vi "Read Page Orientaion.vi"(0 "PdfReader ref":refnum<k24>, 5 "PdfReader page number":i32, 7 "Actual Page number":i32, 9 "Pages dimensions [ ] IN":T1[](array[typedef]) {"Page Size" items=["Custom", "LETTER", "NOTE", "LEGAL", "TABLOID", "EXECUTIVE", "POSTCARD", "A0", "A1", "A2", "A3", "A4", "A5", "A6", "A7", "A8", "A9", "A10", "B0", "B1", "B2", "B3", "B4", "B5", "B6", "B7", "B8", "B9", "B10", "ARCH_E", "ARCH_D", "ARCH_C", "ARCH_B", "ARCH_A", "FLSA", "FLSE", "HALFLETTER", "_11X17", "ID_1", "ID_2", "ID_3", "LEDGER", "CROWN_QUARTO", "LARGE_CROWN_QUARTO", "DEMY_QUARTO", "ROYAL_QUARTO", "CROWN_OCTAVO", "LARGE_CROWN_OCTAVO", "DEMY_OCTAVO", "ROYAL_OCTAVO", "SMALL_PAPERBACK", "PENGUIN_SMALL_PAPERBACK", "PENGUIN_LARGE_PAPERBACK"]}, 11 "error in (no error)":errorcluster) -> (4 "PdfReader ref duplicate":refnum<k24>, 10 "Pages dimensions OUT [ ]":T1[](array[typedef]) {"Page Size" items=["Custom", "LETTER", "NOTE", "LEGAL", "TABLOID", "EXECUTIVE", "POSTCARD", "A0", "A1", "A2", "A3", "A4", "A5", "A6", "A7", "A8", "A9", "A10", "B0", "B1", "B2", "B3", "B4", "B5", "B6", "B7", "B8", "B9", "B10", "ARCH_E", "ARCH_D", "ARCH_C", "ARCH_B", "ARCH_A", "FLSA", "FLSE", "HALFLETTER", "_11X17", "ID_1", "ID_2", "ID_3", "LEDGER", "CROWN_QUARTO", "LARGE_CROWN_QUARTO", "DEMY_QUARTO", "ROYAL_QUARTO", "CROWN_OCTAVO", "LARGE_CROWN_OCTAVO", "DEMY_OCTAVO", "ROYAL_OCTAVO", "SMALL_PAPERBACK", "PENGUIN_SMALL_PAPERBACK", "PENGUIN_LARGE_PAPERBACK"]}, 15 "error out":errorcluster)   [LabVIEW 2019]
doc: "Version 1.1\nDeveloped by Jean-Marc Simard\nCopyright © 2012, Exaprom Inc.\nAll rights reserved.\nLicense: BSD\n\nWith iTextSharp 4.1.6 (http://itextsharp.sourceforge.net)\nunder Mozilla Public License Version 1.1\n(http://www.mozilla.org/MPL/MPL-1.1.html)"
uses:
  <userlib>/Exaprom PDF/Controls/Page Controls/Page dimensions.ctl
  <userlib>/Exaprom PDF/Controls/Page Controls/Page size.ctl
  <userlib>/Exaprom PDF/Controls/Page Controls/Page Orientation.ctl
  C:/Program Files/National Instruments/LabVIEW 2019/user.lib/Exaprom PDF/DLL/itextsharp.dll
  DLL/itextsharp.dll
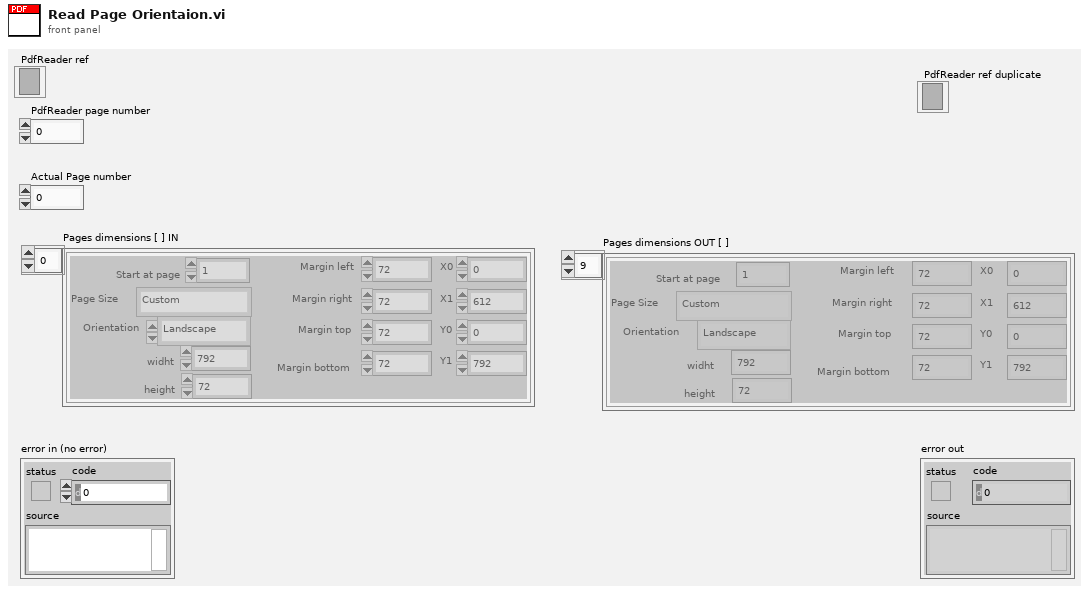
[diagram p1: front panel]
types:
  T1 = typedef "Page dimensions.ctl" = cluster{"Start at page":i32, "Page Size":T2, "Orientation":T3, "widht":sgl, "height":sgl, "Margin left":sgl, "Margin right":sgl, "Margin top":sgl, "Margin bottom":sgl, "X0":sgl, "X1":sgl, "Y0":sgl, "Y1":sgl}
  T2 = typedef "Page size.ctl" = i32
  T3 = typedef "Page Orientation.ctl" = enum16{"Portrait", "Landscape"}
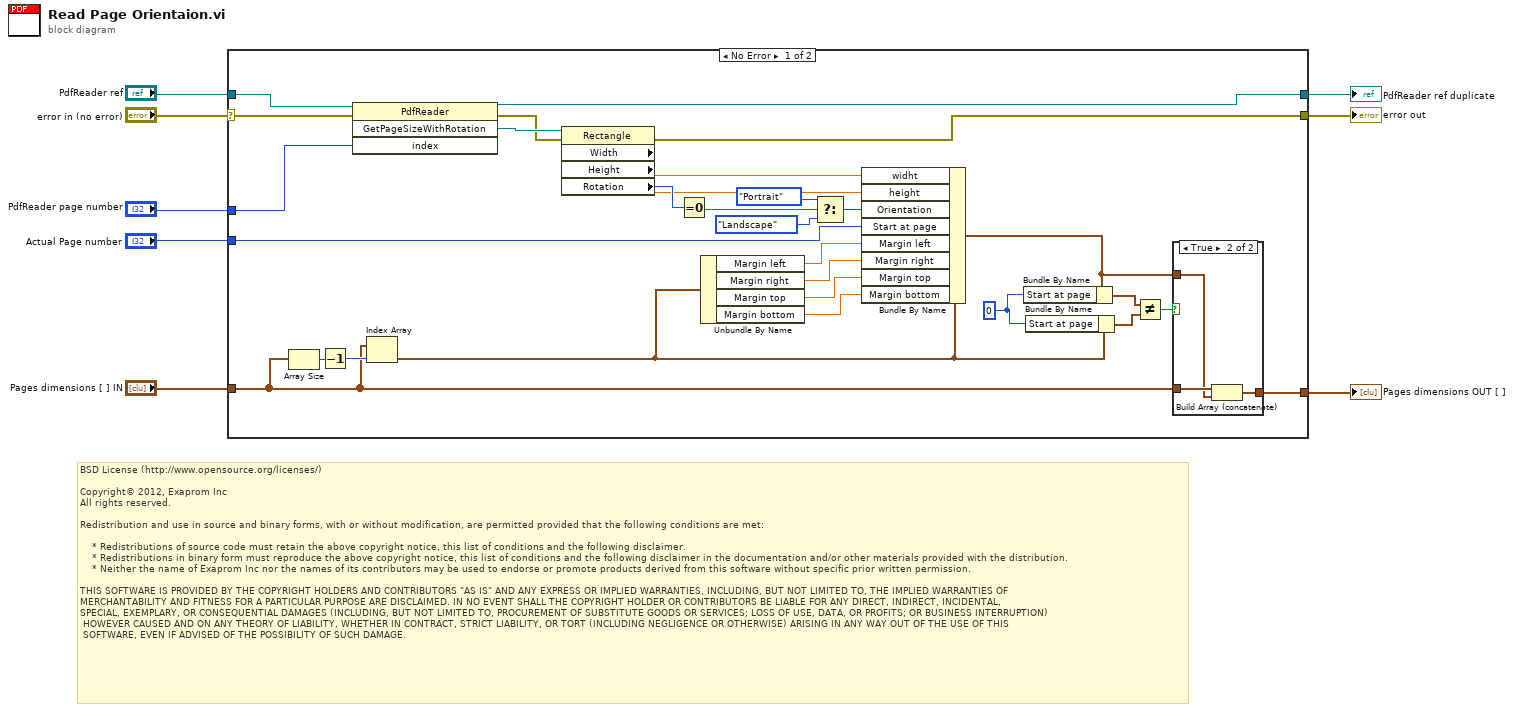
[diagram p0: block diagram]
diagram:
  # "BSD License (http://www.opensource.org/licenses/)\n\nCopyright© 2012, Exaprom Inc\nAll rights reserved.\n\nRedistribution and use in source and binary forms, with or without modification, are permitted provided that the following conditions are met:\n\n    * Redistributions of source code must retain the above copyright notice, this list of conditions and the following disclaimer.\n    * Redistributions in binary form must reproduce the above copyright notice, this list of conditions and the following disclaimer in the documentation and/or other materials provided with the distribution.\n    * Neither the name of Exaprom Inc nor the names of its contributors may be used to endorse or promote products derived from this software without specific prior written permission.\n\nTHIS SOFTWARE IS PROVIDED BY THE COPYRIGHT HOLDERS AND CONTRIBUTORS \"AS IS\" AND ANY EXPRESS OR IMPLIED WARRANTIES, INCLUDING, BUT NOT LIMITED TO, THE IMPLIED WARRANTIES OF \nMERCHANTABILITY AND FITNESS FOR A PARTICULAR PURPOSE ARE DISCLAIMED. IN NO EVENT SHALL THE COPYRIGHT HOLDER OR CONTRIBUTORS BE LIABLE FOR ANY DIRECT, INDIRECT, INCIDENTAL,\nSPECIAL, EXEMPLARY, OR CONSEQUENTIAL DAMAGES (INCLUDING, BUT NOT LIMITED TO, PROCUREMENT OF SUBSTITUTE GOODS OR SERVICES; LOSS OF USE, DATA, OR PROFITS; OR BUSINESS INTERRUPTION)\n HOWEVER CAUSED AND ON ANY THEORY OF LIABILITY, WHETHER IN CONTRACT, STRICT LIABILITY, OR TORT (INCLUDING NEGLIGENCE OR OTHERWISE) ARISING IN ANY WAY OUT OF THE USE OF THIS\n SOFTWARE, EVEN IF ADVISED OF THE POSSIBILITY OF SUCH DAMAGE."
  n1 = case shown="No Error" "error in (no error)" {
    selector: "error in (no error)" -> [w16 w44]
    tunnel: [w15 w44] -> w8
    tunnel: [w14 w42] -> w6
    tunnel: [w13 w43] -> w5
    tunnel: "Pages dimensions [ ] IN" -> [w12 w42]
    tunnel: "Actual Page number" -> [w11 _]
    tunnel: "PdfReader page number" -> [w10 _]
    tunnel: "PdfReader ref" -> [w9 w43]
    frame No Error {
      w30 = 0
      n2 = Array Size(array=w12) -> (size(s)=w36:i32)
      n3 = Decrement(x=w36) -> (x-1=w35:i32)
      n4 = invoke class="PdfReader" method="GetPageSizeWithRotation"(reference=w9, error in=w16, "index"=w10) -> (reference out=w13:refnum<k24>, error out=w17:errorcluster, "GetPageSizeWithRotation"=w18:refnum<k24>)  [unwired: 1 in, 1 out]
      n5 = Index Array(array=w12, index=w35) -> (element=w37:T1)
      n6 = property class="Rectangle"(reference=w18, error in=w17) -> (error out=w15:errorcluster, "Width"=w19:sgl, "Height"=w20:sgl, "Rotation"=w21:i32)  [unwired: 1 out]
      n7 = Equal To 0?(x=w21) -> (x = 0?=w22:bool)
      n8 = Unbundle By Name(w37) -> ("Margin left"=w26:sgl, "Margin right"=w27:sgl, "Margin top"=w28:sgl, "Margin bottom"=w29:sgl)
      n9 = Select(t=Page_Orientation."Portrait" ("Orientation"), s=w22, f=Page_Orientation."Landscape" ("Orientation")) -> (s? t:f=w25:T3)
      n10 = Bundle By Name(cluster=w37, "widht"=w19, "height"=w20, "Orientation"=w25, "Start at page"=w11, "Margin left"=w26, "Margin right"=w27, "Margin top"=w28, "Margin bottom"=w29) -> (w34:T1)
      n11 = Bundle By Name(cluster=w34, "Start at page"=w30) -> (w31:T1)
      n12 = Bundle By Name(cluster=w37, "Start at page"=w30) -> (w32:T1)
      n13 = Not Equal?(x=w31, y=w32) -> (x != y?=w33:bool)
      n14 = case shown="True" w33 {
        tunnel: w12 -> [w38 w41]
        tunnel: [w38 w40] -> w14
        tunnel: w34 -> [_ w39]
        frame False {
        }
        frame True {
          n15 = Build Array (concatenate)(w41, w39) -> (w40:T1[])
        }
      }
    }
    frame Error {
    }
  }
  "error out" <- w8
  "Pages dimensions OUT [ ]" <- w6
  "PdfReader ref duplicate" <- w5
